vi "QMgr_EnQueue.vi"(7 "Data":variant, 10 "Command":string, 11 "queue in":refnum<queue>) -> (3 "queue out":refnum<queue>)   [LabVIEW 2016, in "MB Master.lvlib" / "MB_Master_TCP.lvclass"]
uses:
  MB_Master_TCP.lvclass
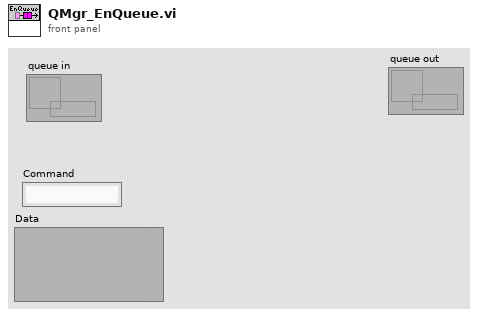
[diagram p1: front panel]
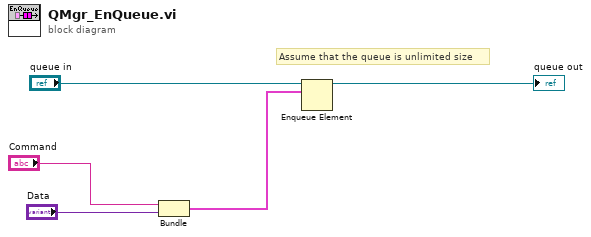
[diagram p0: block diagram]
diagram:
  # "Assume that the queue is unlimited size"
  n1 = Bundle("Command"="Command", "Data"="Data") -> (w2:cluster{"Command":string, "Data":variant})  [unwired: 1 in]
  n2 = Enqueue Element(queue="queue in", element=w2) -> (queue out=→"queue out":refnum<queue>)  [unwired: 2 in, 2 out]
